vi "2 curves in single plot.vi"() -> ()   [LabVIEW 2017]
panel:
  in  "Y2":dbl[](array[numeric])=[3.0, 4.0, 2.0]
  in  "X2":dbl[](array[numeric])=[0.5, 1.5, 3.5]
  in  "Y1":dbl[](array[numeric])=[2.0, 1.0, 0.0]
  in  "X1":dbl[](array[numeric])=[1.0, 2.0, 4.0]
  out "XY Graph":cluster{dbl[], dbl[]}[](graph)=[{[1.0, 2.0, 4.0], [2.0, 1.0, 0.0]}, {[0.5, 1.5, 3.5], [3.0, 4.0, 2.0]}]
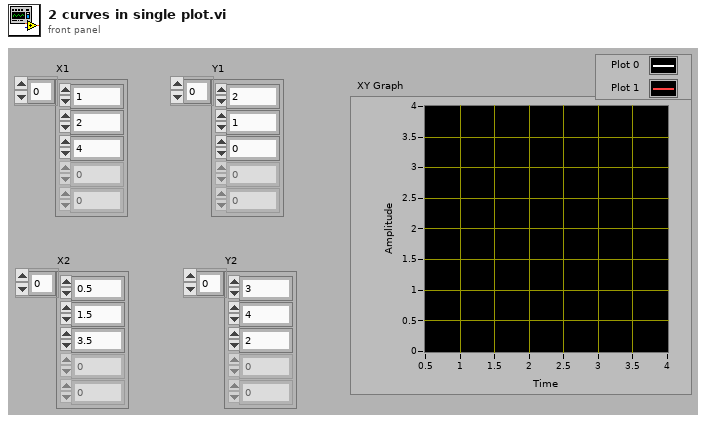
[diagram p1: front panel]
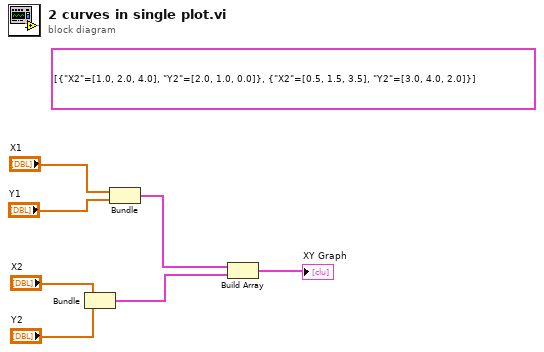
[diagram p0: block diagram]
diagram:
  (unwired) cluster{"X2":dbl[], "Y2":dbl[]}[] [{"X2"=[1.0, 2.0, 4.0], "Y2"=[2.0, 1.0, 0.0]}, {"X2"=[0.5, 1.5, 3.5], "Y2"=[3.0, 4.0, 2.0]}] ("appended array")
  n1 = Bundle("X2"="X2", "Y2"="Y2") -> (w2:cluster{"X2":dbl[], "Y2":dbl[]})  [unwired: 1 in]
  n2 = Bundle("X1"="X1", "Y1"="Y1") -> (w3:cluster{"X1":dbl[], "Y1":dbl[]})  [unwired: 1 in]
  n3 = Build Array(w3, w2) -> (→"XY Graph":cluster{"X2":dbl[], "Y2":dbl[]}[])
